vi "Tree Group Parsing.vi"() -> ()   [LabVIEW 2019]
panel:
  out "array of clusters":T1(array[cluster])
  in  "XML":string
  out "Array":cluster{"Start":i32, "data":string, "End":i32}[](array[cluster])
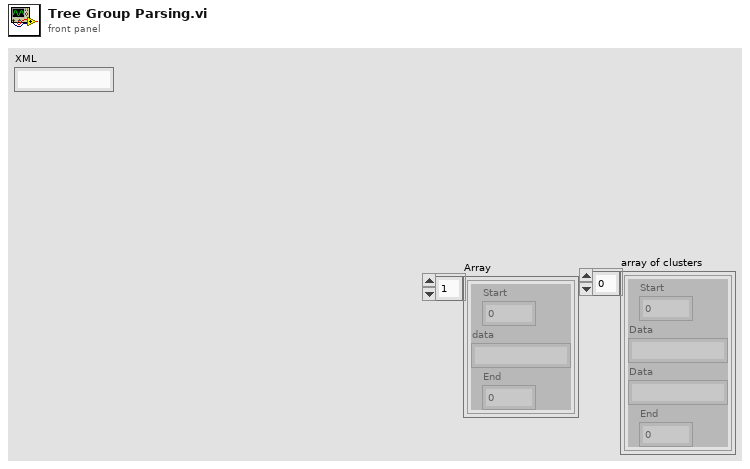
[diagram p1: front panel]
types:
  T1 = cluster{"Start":i32, "Data":string, "Data":string, "End":i32}[]
  T2 = cluster{"Start":i32, "id":string, "transforms":string, "End":i32}[]
  T3 = cluster{"offset past match":i32, "RawXML":string}
  T4 = cluster{"offset past match":i32, "RawXML":string}[]
  T5 = cluster{"offset past match":i32, "regular expression":string}[]
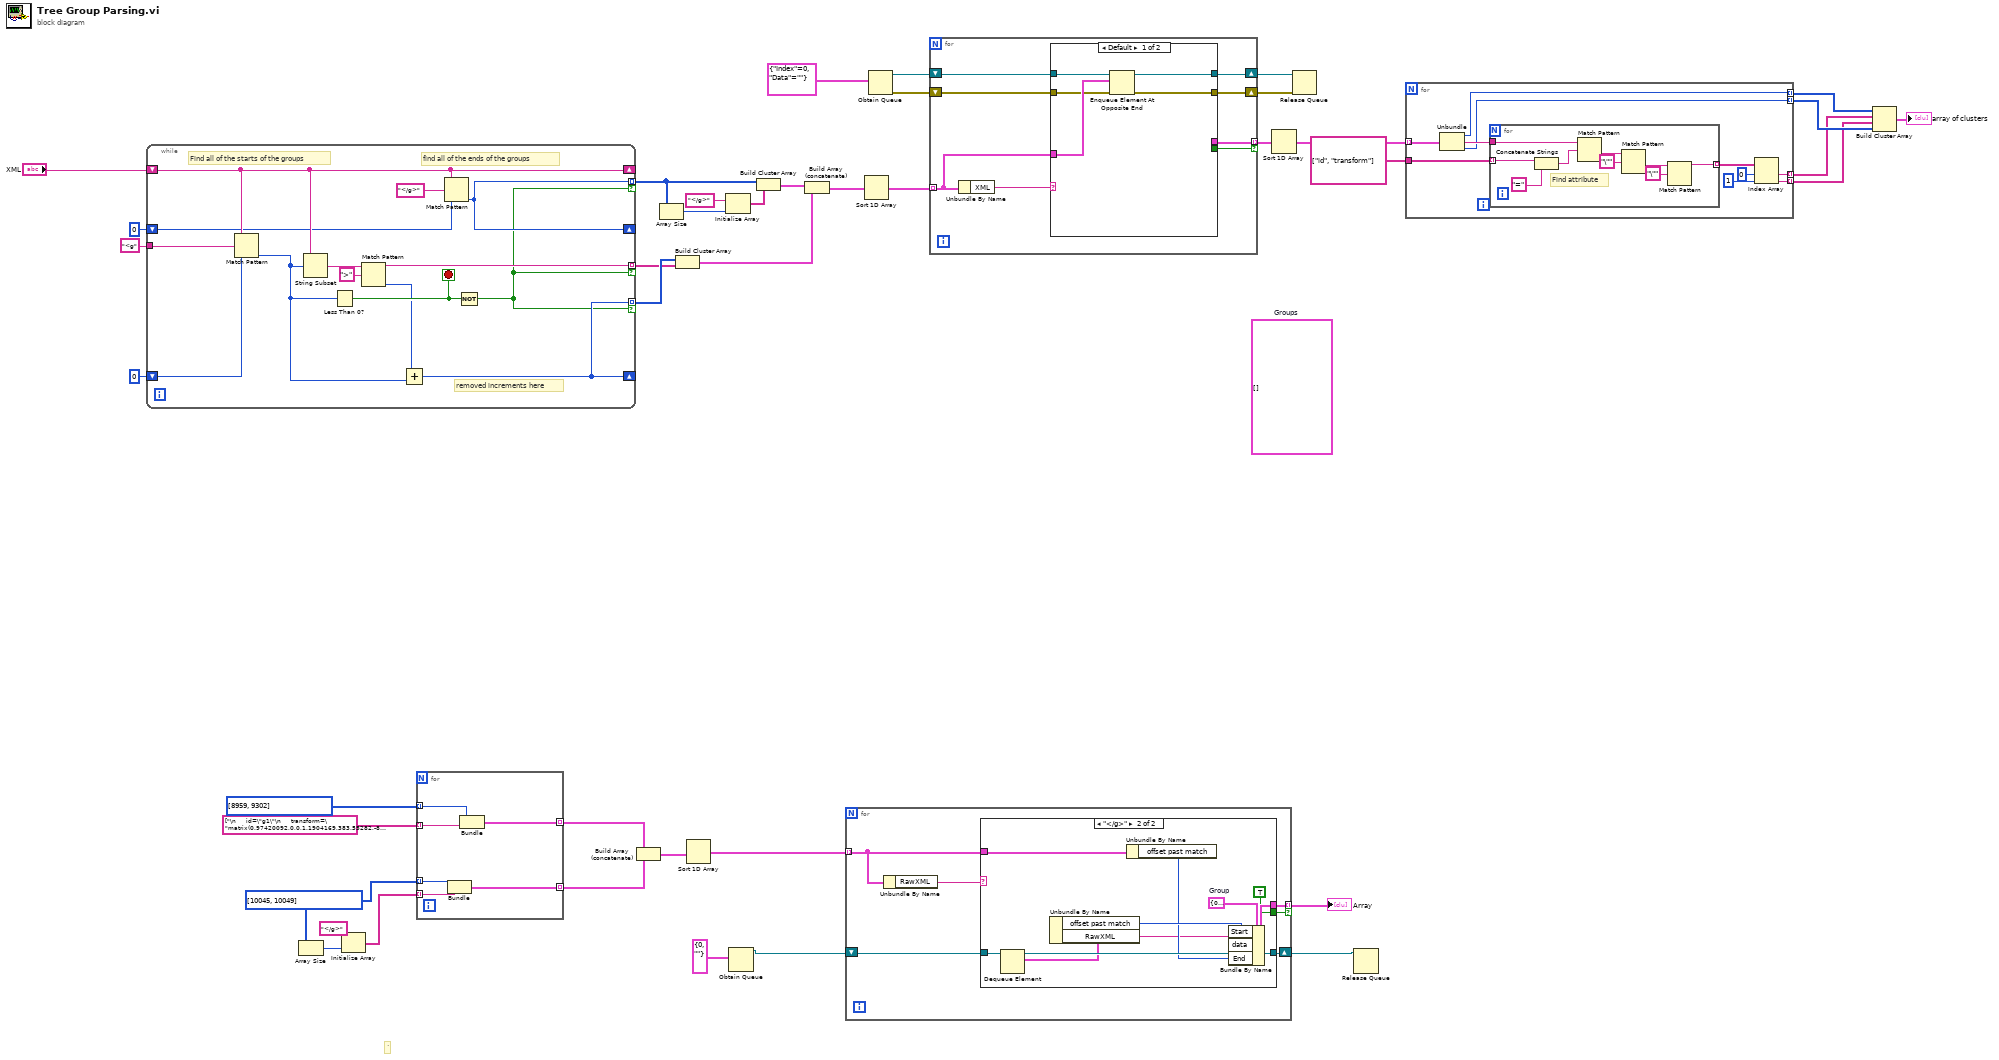
[diagram p0: block diagram]
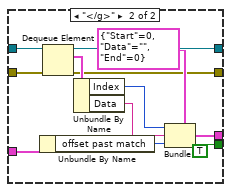
[diagram p2: hidden frame]
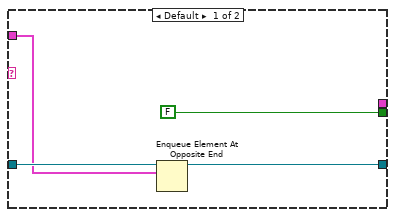
[diagram p3: hidden frame]
diagram:
  (unwired) T2 []  # Groups
  w36 = i32[] [10045, 10049] ("reversed array")
  # "`"
  n1 = while {
    shift-right: [w50] -> _
    shift-left: "XML" -> [w50]
    shift-right: [w45] -> _
    shift-left: 0 -> [w54]
    tunnel: [w44] -> w12 mode=indexing if=w42
    tunnel: "<g" -> [w47]
    tunnel: [w43] -> w5 mode=indexing if=w42
    tunnel: [w45] -> w18 mode=indexing if=w42
    shift-right: [w43] -> _
    shift-left: 0 ("offset past match") -> [w46]
    stop <- w52 stop-if-true
    # "removed increments here"
    # "Find all of the starts of the groups"
    # "find all of the ends of the groups"
    n2 = Match Pattern(string=w50, regular expression=w47, offset (0)=w54) -> (offset past match=w48:i32)  [unwired: 3 out]
    n3 = String Subset(string=w50, offset (0)=w48) -> (substring=w55:string)  [unwired: 1 in]
    n4 = Less Than 0?(x=w48) -> (x < 0?=w52:bool)
    n5 = Match Pattern(string=w55, regular expression=">") -> (before substring=w44:string, offset past match=w51:i32)  [unwired: 1 in, 2 out]
    n6 = Add(x=w51, y=w48) -> (x+y=w45:i32)
    n7 = Match Pattern(string=w50, regular expression="</g>", offset (0)=w46) -> (offset past match=w43:i32)  [unwired: 3 out]
    n8 = Not(x=w52) -> (.not. x?=w42:bool)
  }
  n9 = Array Size(array=w36) -> (size(s)=w39:i32)
  n10 = Initialize Array("</g>", w39) -> (w37:string[])
  n11 = for {
    tunnel: i32[] [8959, 9302] ("Array") -> [w61] mode=indexing
    tunnel: string[] ["\n     id=\"g1\"\n     transform=\"matrix(0.97420092,0,0,1.1904169,383.55282,-892.60137)\"", "\n       id=\"g3\"\n       transform=\"matrix(0.87240932,-0.1215228,0.11425413,0.92791062,3276.3322,3478.6107)\""] ("Array 2") -> [w60] mode=indexing
    tunnel: w37 -> [w58] mode=indexing
    tunnel: w36 -> [w59] mode=indexing
    tunnel: [w57] -> w34 mode=indexing
    tunnel: [w56] -> w35 mode=indexing
    n12 = Bundle("offset past match"=w59, w58) -> (w57:cluster{"offset past match":i32, string})  [unwired: 1 in]
    n13 = Bundle(w61, "RawXML"=w60) -> (w56:cluster{i32, "RawXML":string})  [unwired: 1 in]
  }
  n14 = Build Array (concatenate)(w35, w34) -> (w33:T4)
  n15 = Array Size(array=w5) -> (size(s)=w17:i32)
  n16 = Build Cluster Array(w18, w12) -> (w14:cluster{i32, "XML":string}[])
  n17 = Sort 1D Array(array=w33) -> (sorted array=w31:T4)
  n18 = Initialize Array("</g>" ("regular expression"), w17) -> (w15:string[])
  n19 = Obtain Queue(element data type=T3 {"offset past match"=0, "RawXML"=""}) -> (queue out=w30:refnum<queue>)  [unwired: 4 in, 2 out]
  n20 = Build Cluster Array(w5, w15) -> (w4:T5)
  n21 = Build Array (concatenate)(w4, w14) -> (w13:cluster{"offset past match":i32, "XML":string}[])
  n22 = for {
    tunnel: w31 -> [w66] mode=indexing
    shift-right: [w64] -> w28
    shift-left: w30 -> [w65]
    tunnel: [w63] -> w29 mode=indexing if=w62
    n23 = Unbundle By Name(w66) -> ("RawXML"=w67:string)
    n24 = case shown="\"</g>\"" w67 {
      tunnel: w66 -> [w69 w79]
      tunnel: w65 -> [w71 w81]
      tunnel: [w70 w80] -> w64
      tunnel: [_ w73] -> w63
      tunnel: [FALSE TRUE] -> w62
      frame Default {
        n25 = Enqueue Element At Opposite End(queue=w71, element=w69) -> (queue out=w70:refnum<queue>)  [unwired: 2 in, 2 out]
      }
      frame "</g>" {
        w78 = cluster{"Start":i32, "data":string, "End":i32} {"Start"=0, "data"="", "End"=0}  # Group
        n26 = Dequeue Element(queue=w81) -> (queue out=w80:refnum<queue>, element=w77:T3)  [unwired: 2 in, 2 out]
        n27 = Unbundle By Name(w77) -> ("offset past match"=w76:i32, "RawXML"=w74:string)
        n28 = Unbundle By Name(w79) -> ("offset past match"=w75:i32)
        n29 = Bundle By Name(cluster=w78, "Start"=w76, "data"=w74, "End"=w75) -> (w73:cluster{"Start":i32, "data":string, "End":i32})
      }
    }
  }
  "Array" <- w29
  n30 = Sort 1D Array(array=w13) -> (sorted array=w20:cluster{"offset past match":i32, "XML":string}[])
  n31 = Obtain Queue(element data type=cluster{"Index":i32, "Data":string} {"Index"=0, "Data"=""}) -> (queue out=w21:refnum<queue>, error out=w2:errorcluster)  [unwired: 4 in, 1 out]
  n32 = for {
    tunnel: w20 -> [w88] mode=indexing
    shift-right: [w87] -> w3
    shift-left: w21 -> [w86]
    tunnel: [w85] -> w19 mode=indexing if=w84
    shift-right: [w82] -> w1
    shift-left: w2 -> [w83]
    n33 = Unbundle By Name(w88) -> ("XML"=w89:string)
    n34 = case shown="Default" w89 {
      tunnel: w88 -> [w92 w103]
      tunnel: [w94 w105] -> w87
      tunnel: w86 -> [w93 w106]
      tunnel: [_ w98] -> w85
      tunnel: [_ TRUE] -> w84
      tunnel: w83 -> [w91 w96]
      tunnel: [w90 w95] -> w82
      frame Default {
        n35 = Enqueue Element At Opposite End(queue=w93, element=w92, error in (no error)=w91) -> (queue out=w94:refnum<queue>, error out=w90:errorcluster)  [unwired: 1 in, 1 out]
      }
      frame "</g>" {
        n36 = Unbundle By Name(w103) -> ("offset past match"=w99:i32)
        n37 = Dequeue Element(queue=w106, error in (no error)=w96) -> (queue out=w105:refnum<queue>, element=w104:cluster{"Index":i32, "Data":string}, error out=w95:errorcluster)  [unwired: 1 in, 1 out]
        n38 = Unbundle By Name(w104) -> ("Index"=w101:i32, "Data"=w100:string)
        n39 = Bundle(cluster=cluster{"Start":i32, "Data":string, "End":i32} {"Start"=0, "Data"="", "End"=0}, "Start"=w101, "Data"=w100, "End"=w99) -> (w98:cluster{"Start":i32, "Data":string, "End":i32})
      }
    }
  }
  n40 = Sort 1D Array(array=w19) -> (sorted array=w11:cluster{"Start":i32, "Data":string, "End":i32}[])
  n41 = Release Queue(queue=w3, error in (no error)=w1) -> ()  [unwired: 1 in, 3 out]
  n42 = Release Queue(queue=w28) -> ()  [unwired: 2 in, 3 out]
  n43 = for {
    tunnel: w11 -> [w109] mode=indexing
    tunnel: string[] ["id", "transform"] -> [w116]
    tunnel: [w112] -> w8 mode=indexing
    tunnel: [w111] -> w7 mode=indexing
    tunnel: [w108] -> w10 mode=indexing
    tunnel: [w107] -> w9 mode=indexing
    n44 = Unbundle(w109) -> ("Start"=w108:i32, "Data"=w110:string, "End"=w107:i32)
    n45 = for {
      tunnel: w110 -> [w125]
      tunnel: w116 -> [w118] mode=indexing
      tunnel: [w117] -> w115 mode=indexing
      # "Find attribute"
      n46 = Concatenate Strings(w118, "=" ("string")) -> (w120:string)
      n47 = Match Pattern(string=w125, regular expression=w120) -> (after substring=w124:string)  [unwired: 1 in, 3 out]
      n48 = Match Pattern(string=w124, regular expression="\"") -> (after substring=w122:string)  [unwired: 1 in, 3 out]
      n49 = Match Pattern(string=w122, regular expression="\"") -> (before substring=w117:string)  [unwired: 1 in, 3 out]
    }
    n50 = Index Array(array=w115, index #1=0 ("index"), index #2=1 ("index")) -> (element #1=w112:string, element #2=w111:string)
  }
  n51 = Build Cluster Array(w10, w8, w7, w9) -> (→"array of clusters":T1)
